vi "findphi+theta.vi"(9 "Final Distance away from the target To stop at":dbl=4.0 format="%#_13g", 11 "Vision Angle  difference from target":dbl format="%#_13g") -> ()   [LabVIEW 2018]
panel:
  in  "Vision distance from target":dbl=4.0 format="%#_13g"
  out "Gyro Setpoint B":dbl format="%#_13g"
  out "Encoders Setpoint to drive":dbl format="%#_13g"
  out "Gyro Setpoint A":dbl format="%#_13g"
  in  "Current Gyro":dbl=4.0 format="%#_13g"
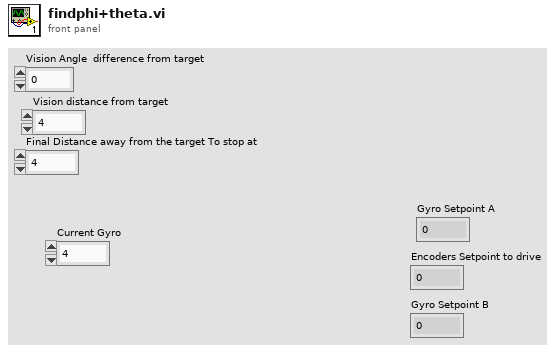
[diagram p1: front panel]
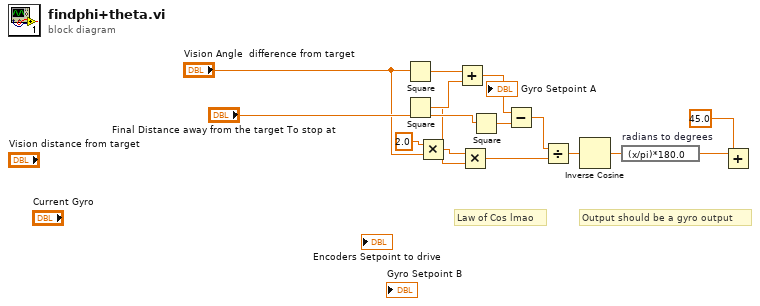
[diagram p0: block diagram]
diagram:
  # "Output should be a gyro output"
  # "Law of Cos lmao"
  n1 = Square(x="Vision Angle  difference from target") -> (x^2=w16:dbl)
  n2 = Square() -> (x=w7:dbl, x^2=w15:dbl)
  n3 = Multiply(x=2.0, y="Vision Angle  difference from target") -> (x*y=w8:dbl)
  n4 = Add(x=w16, y=w15) -> (x+y=w14:dbl)
  n5 = Multiply(x=w8, y=w7) -> (x*y=w6:dbl)
  n6 = Square(x="Final Distance away from the target To stop at") -> (x^2=w12:dbl)
  n7 = Subtract(x=w14, y=w12) -> (x-y=w11:dbl)
  n8 = Divide(x=w11, y=w6) -> (x/y=w5:dbl)
  n9 = Inverse Cosine(1:w5) -> (0:w4:dbl)
  n10 = expression code="(x/pi)*180.0" "radians to degrees"(w4) -> (w3:dbl)
  n11 = Add(x=w3, y=45.0) -> (x+y=w1:dbl)
